vi "hasPacketIdentifier.vi"(11 "PUBREC in":refnum<class "PUBREC.lvclass">) -> (2 "Has Packet Identifier":bool, 3 "PUBREC out":refnum<class "PUBREC.lvclass">)   [LabVIEW 2013, in "MQTT_Control_Packets.lvlib" / "PUBREC.lvclass"]
uses:
  PUBREC.lvclass
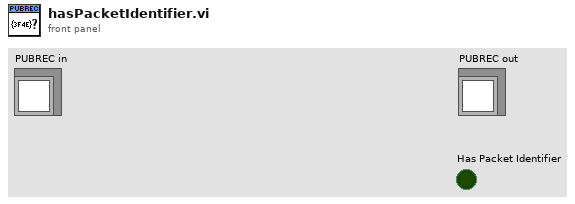
[diagram p1: front panel]
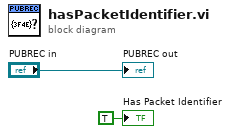
[diagram p0: block diagram]
diagram:
  "PUBREC out" <- "PUBREC in"
  "Has Packet Identifier" <- TRUE ("As Packet Identifier")
